vi "FIB trapezoidal mill PXIe-6124.vi"(0 "ActiveX Container":refnum<k7>(container), 1 "COM port":refnum<visa-resource-name>="COM1", 3 "WatchDog Mode":u16(ring)=2 items=["Do Nothing", "Send Idle Only", "Watch FIB & SEM", "Watch FIB Only", "Watch SEM Only"], 5 "FIB Scan Parameters":T3={"X resolution"=512, "Z resolution"=512, "X center"=0.0, "Z center"=0.0, "X size (V)"=20.0, "Z size (V)"=20.0, "Frame line rampdown ratio"=-0.1, "Scan rate (Hz)"=2000000, "Oversampling"=2} {"Z size (V)" min=0.0 max=20.0; "X size (V)" min=0.0 max=20.0; "Frame line rampdown ratio" min=-1.0 max=1.0 step=0.05 format="%.2g"; "Scan rate (Hz)" max=4000000 format="%#.6p"; "Z resolution" max=2048; "X resolution" max=2048}, 7 "FIB HW Config":T4={"FIB X coil"="FIB/ao0", "FIB Y coil"="FIB/ao1", "Beam blank"="FIB/port0/line0", "Ext scan"="FIB/port0/line1", "Detector"="FIB/ai0", "Shutter Drive"="Log/ao0"}, 9 "Options":cluster{"Flip x":bool, "Flip z":bool}={"Flip x"=TRUE, "Flip z"=TRUE}, 11 "Milling para":T1={"X resolution"=4096, "Z resolution"=125001, "X offset (um)"=0.0, "Z offset (um)"=0.0, "X center (um)"=0.0, "Z center (um)"=0.0, "X size (um)"=250.0, "Z size (um)"=250.0, "UL-Ang"=90.0, "UR-Ang"=90.0, "Line milling time (s)"=5.0, "Z-step (nm)"=2.0, "Lines auto pause"=1, "Auto pause"=FALSE, "Mill from Bottom"=FALSE, "FIB FOV (um)"=500.0, "Auto Profile"=FALSE, "Mill start from Last"=FALSE, "FIB PID on"=FALSE, "FIB PID reset"=TRUE, "FIB PID measured"=0, "FIB PID target"=0.0, "FIB PID target slope"=0.0, "FIB PID P"=0.001, "FIB PID I"=0.01, "FIB PID D"=0.0, "Emission (uA)"=1.36, "Suppressor (V)"=50.0, "Auto reheat"=FALSE} caption="Milling Parameters" {"Suppressor (V)" step=0.1 format="%.1g"; "Emission (uA)" step=0.1 format="%.2g"; "FIB PID measured" items=["Spec.", "B.D. 1", "B.D. 2", "Mill", "Spec. +"]; "FIB PID target slope" min=-1 max=1 step=0.1; "UR-Ang" format="%.2f"; "UL-Ang" format="%.2f"; "Z offset (um)" step=0.02 format="%.3g"; "X offset (um)" step=1 format="%.3g"; "FIB FOV (um)" format="%.3g"; "Line milling time (s)" format="%.1f"; "Z center (um)" format="%#.3g"; "X center (um)" format="%#.3g"}, 12 "Machine Type":u8(ring) items=["Feiss", "NVision", "Jeiss"], 14 "Damping":bool) -> (4 "Line progress":u8(slide) scale=0.0..100.0, 6 "Total progress":u8(slide) scale=0.0..100.0, 10 "post-pause lines":u16, 15 "error out":errorcluster)   [LabVIEW 2018]
uses:
  <vilib>/DAQmx/write.llb/DAQmx Write (Analog 2D DBL NChan NSamp).vi
  <vilib>/DAQmx/write.llb/DAQmx Write (Analog 1D DBL 1Chan NSamp).vi
  <vilib>/Analysis/baseanly.llb/Mean (DBL).vi
  <vilib>/DAQmx/write.llb/DAQmx Write (Analog DBL 1Chan 1Samp).vi
  <vilib>/DAQmx/write.llb/DAQmx Write (Analog 1D DBL NChan 1Samp).vi
  <vilib>/DAQmx/create/channels.llb/DAQmx Create Channel (AO-Voltage-Basic).vi
  <vilib>/DAQmx/configure/timing.llb/DAQmx Timing (Sample Clock).vi
  <vilib>/DAQmx/miscellaneous.llb/DAQmx Fill In Error Info.vi
  <vilib>/measure/madcrms.llb/Basic Averaged DC-RMS for 1 Chan.vi
  <vilib>/Analysis/NI_AALBase.lvlib
  <vilib>/measure/NI_MAPro.lvlib
panel:
  out "SEM shutter status":string
  out "Fail #":u8
  out "FIB PID measured":u8
  out "FIB PID on offset":dbl
  out "FIB PID target slope":sgl
  out "FIB PID feedback mean":dbl
  out "FIB PID FB array":dbl[](array[numeric])
  out "Beam blanked":bool=TRUE
  out "FIB PID D":sgl
  out "FIB PID I":sgl
  out "FIB PID P":sgl
  out "FIB PID target":sgl
  out "FIB PID reset":bool
  out "FIB PID on":bool
  out "FIB PID feedback":dbl
  out "UR-Ang":sgl=90.0
  out "UL-Ang":sgl=90.0
  in  "FIB bit size (nm)":dbl
  out "X offset":sgl
  out "Y offset":sgl
  in  "Sweep enabled":bool
  in  "Focus (V)":dbl min=-10.0 max=10.0 step=0.1 format="%.3g"
  in  "Imbalance (V)":dbl min=-10.0 max=10.0 step=0.1 format="%.3f"
  in  "Sweep direction":bool
  in  "Angle (V)":dbl min=-10.0 max=10.0 step=0.1 format="%.3g"
  in  "Position (V)":dbl min=-10.0 max=10.0 step=0.1 format="%.3g"
  in  "Level #":u8
  in  "Sweep #":u8=1 min=1
  out "Shutter Drive":tag="PXI1Slot2/ao0"
  out "Milling mode":T2(ring)=enum."SEM + FIB"
  out "Z voltage RT":dbl
  out "Ext scan":tag="PXI1Slot4/port0/line1"
  out "FIB Y coil":tag="PXI1Slot4/ao1"
  out "FIB X coil":tag="PXI1Slot4/ao0"
  out "Mill from Bottom":bool
  out "Line Paused":bool
  in  "Resume":bool
  in  "Manual pause":bool
  out "Auto pause":bool
  out "Line milling time (s)":sgl=10.0
  out "Lines auto pause":u16=1
  out "Y size":sgl=1.0
  out "X size":sgl=1.0
  out "Y center":sgl
  out "X center":sgl
  out "Y resolution":u32=100
  out "X resolution":u32=16384
  in  "Stop":bool
  out "Beam blank":tag="PXI1Slot4/port0/line0"
  # "% of"
  # "th line"
  # "%"
  # "Direction"
  # "Start\nfrom"
  # "<"
  # "Scan coils"
  # "Flip"
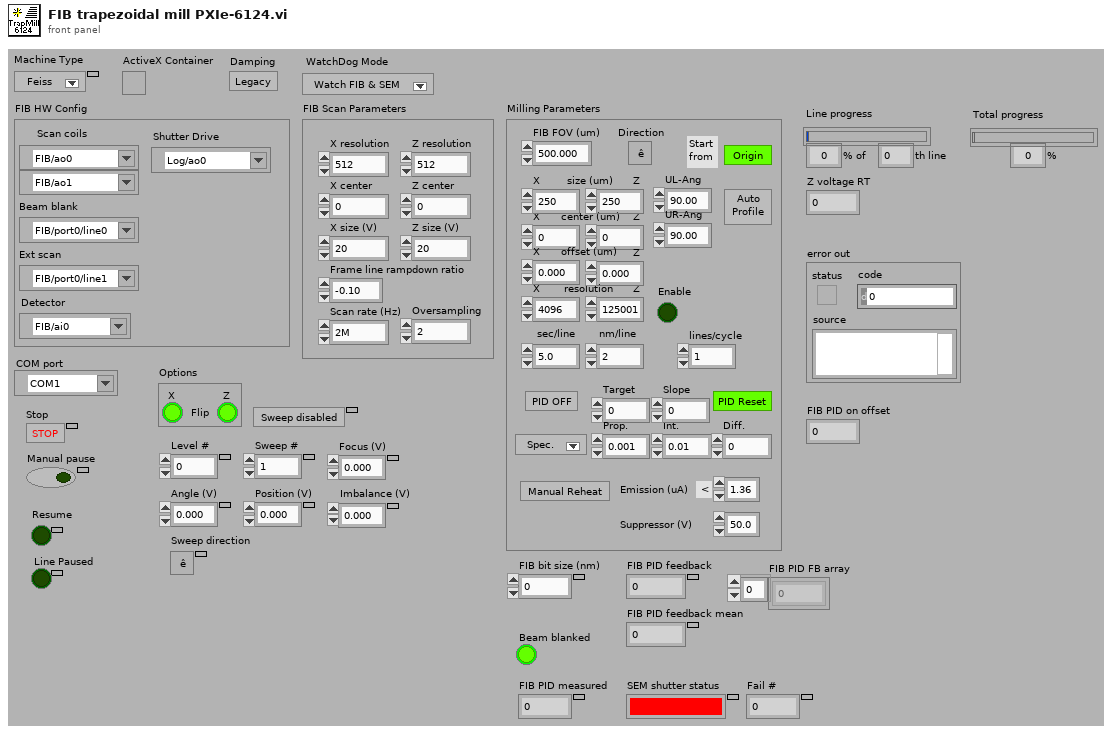
[diagram p1: front panel]
types:
  T1 = cluster{"X resolution":u32, "Z resolution":u32, "X offset (um)":sgl, "Z offset (um)":sgl, "X center (um)":sgl, "Z center (um)":sgl, "X size (um)":sgl, "Z size (um)":sgl, "UL-Ang":sgl, "UR-Ang":sgl, "Line milling time (s)":sgl, "Z-step (nm)":dbl, "Lines auto pause":u16, "Auto pause":bool, "Mill from Bottom":bool, "FIB FOV (um)":sgl, "Auto Profile":bool, "Mill start from Last":bool, "FIB PID on":bool, "FIB PID reset":bool, "FIB PID measured":u8, "FIB PID target":sgl, "FIB PID target slope":sgl, "FIB PID P":sgl, "FIB PID I":sgl, "FIB PID D":sgl, "Emission (uA)":dbl, "Suppressor (V)":sgl, "Auto reheat":bool}
  T2 = enum16{"SEM", "FIB", "Milling", "SEM + FIB", "Mill + SEM", "SEM Drift Correction", "FIB Drift Correction", "No Beam", "External", "External + SEM"}
  T3 = cluster{"X resolution":u32, "Z resolution":u32, "X center":dbl, "Z center":dbl, "X size (V)":dbl, "Z size (V)":dbl, "Frame line rampdown ratio":dbl, "Scan rate (Hz)":u32, "Oversampling":u16}
  T4 = cluster{"FIB X coil":tag, "FIB Y coil":tag, "Beam blank":tag, "Ext scan":tag, "Detector":tag, "Shutter Drive":tag}
  T5 = enum16{"SEM", "FIB", "Mill", "SEM + FIB", "Mill + SEM", "Drift SEM", "Drift FIB", "None", "Ext", "Ext + SEM"}
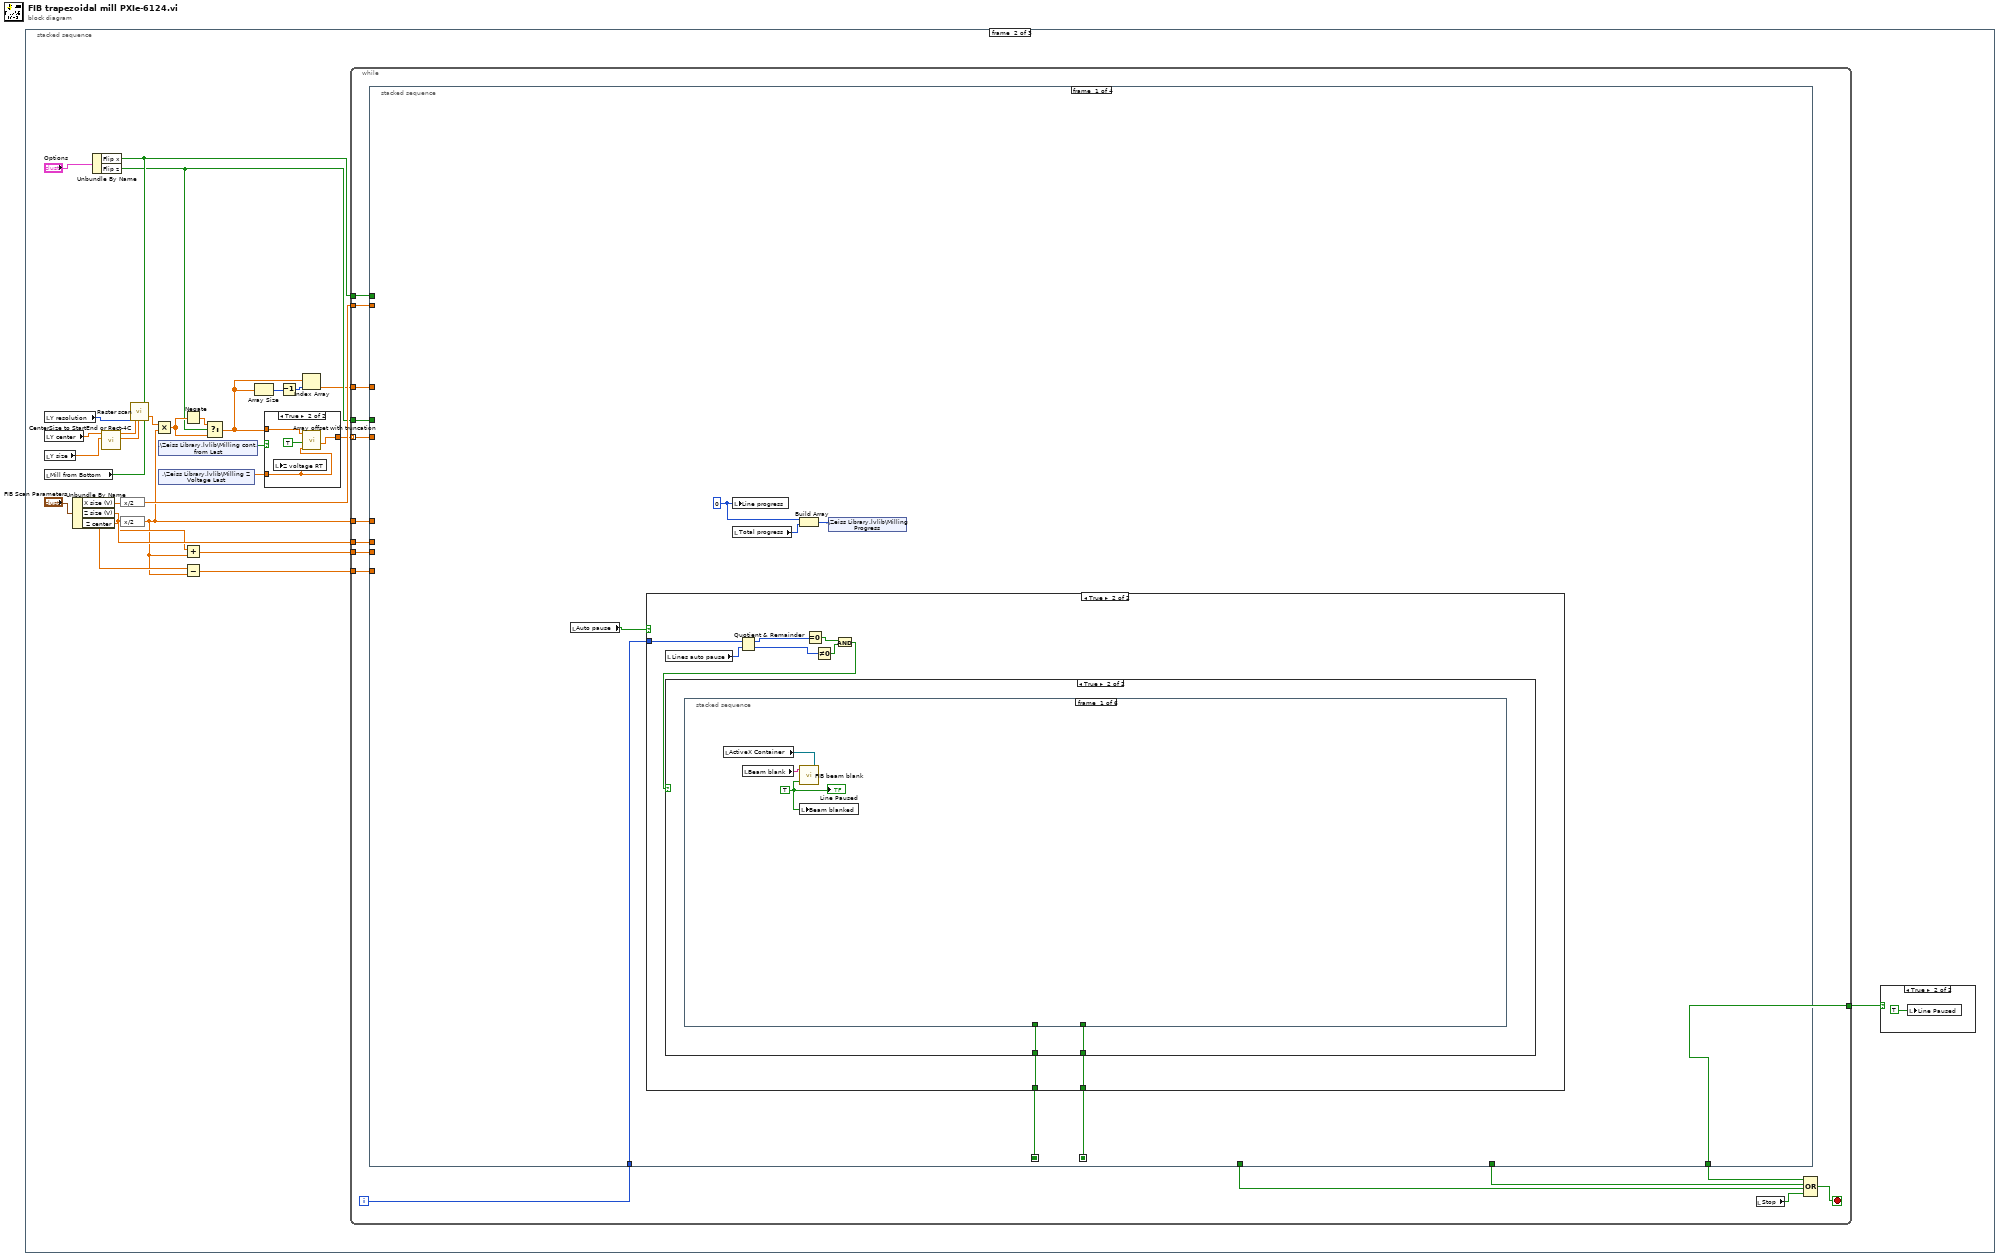
[diagram p0: block diagram]
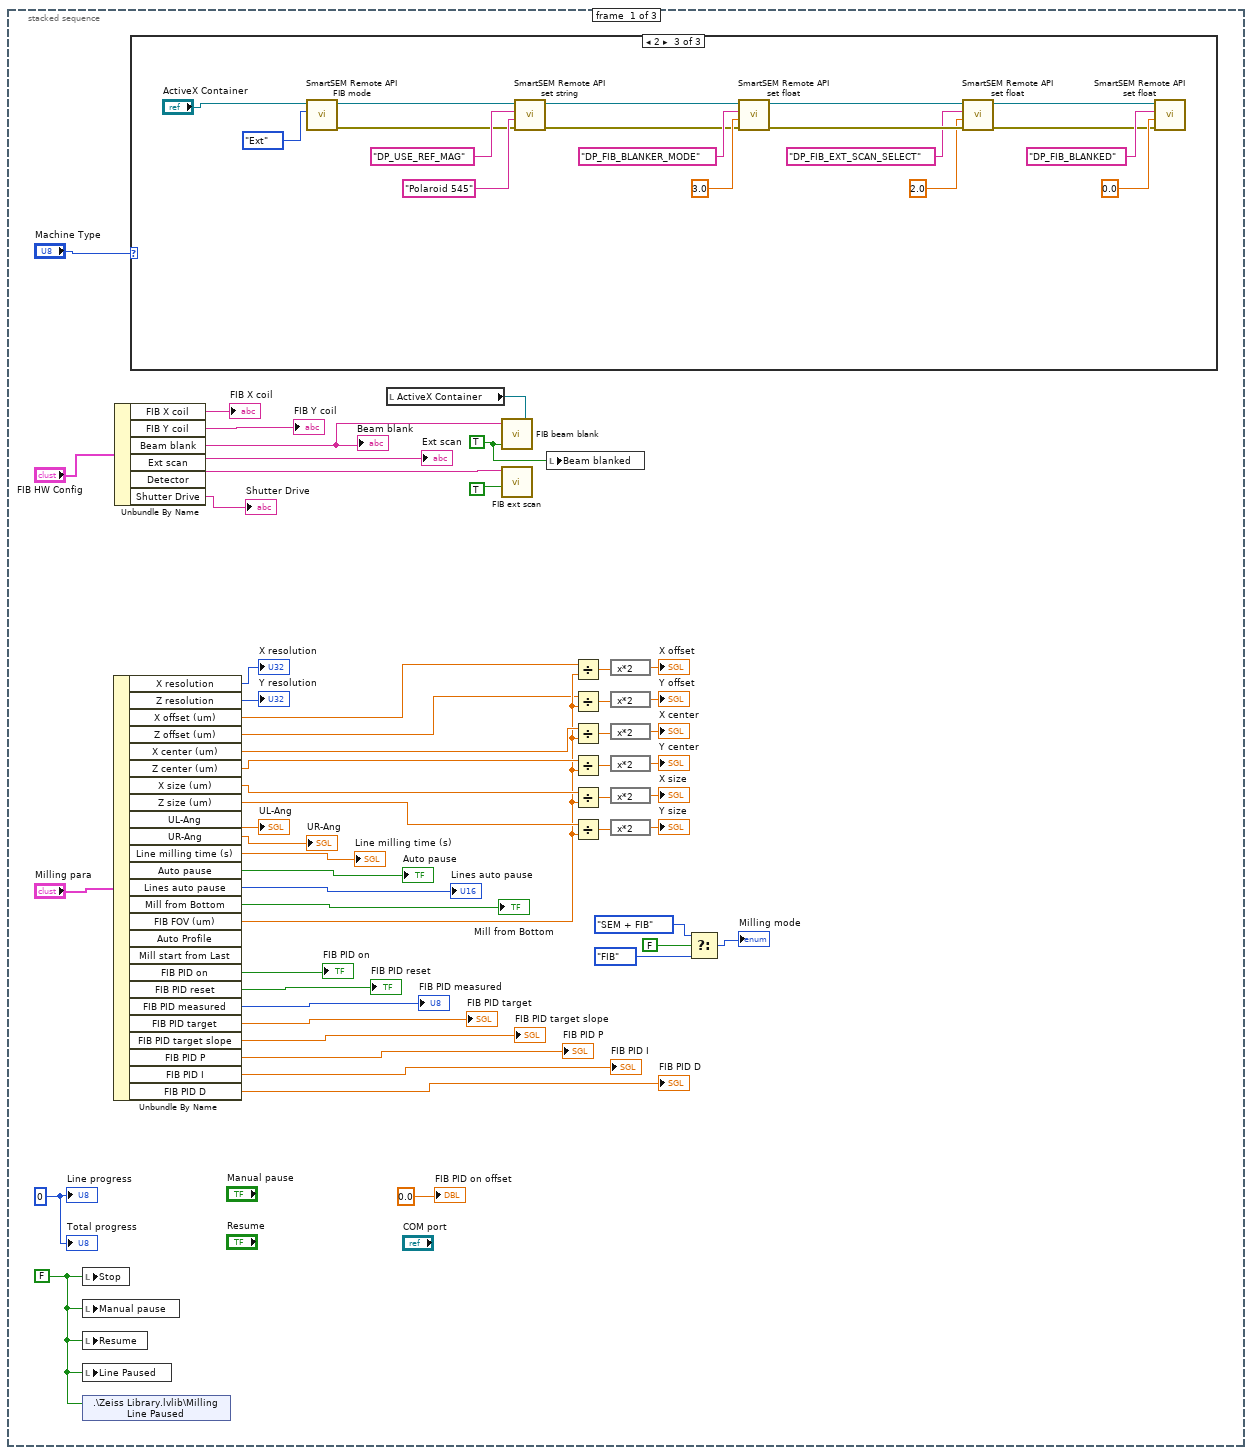
[diagram p2: hidden frame]
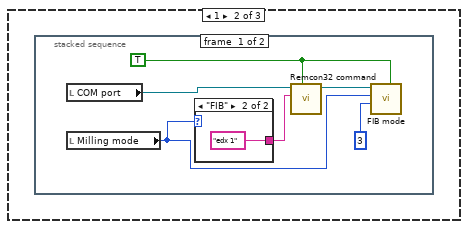
[diagram p4: hidden frame]
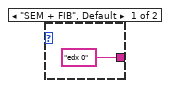
[diagram p5: hidden frame]
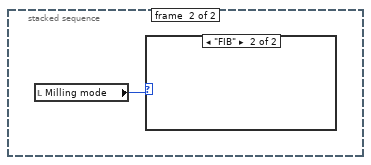
[diagram p6: hidden frame]
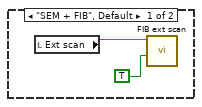
[diagram p7: hidden frame]
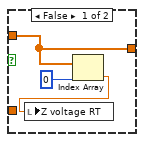
[diagram p8: hidden frame]
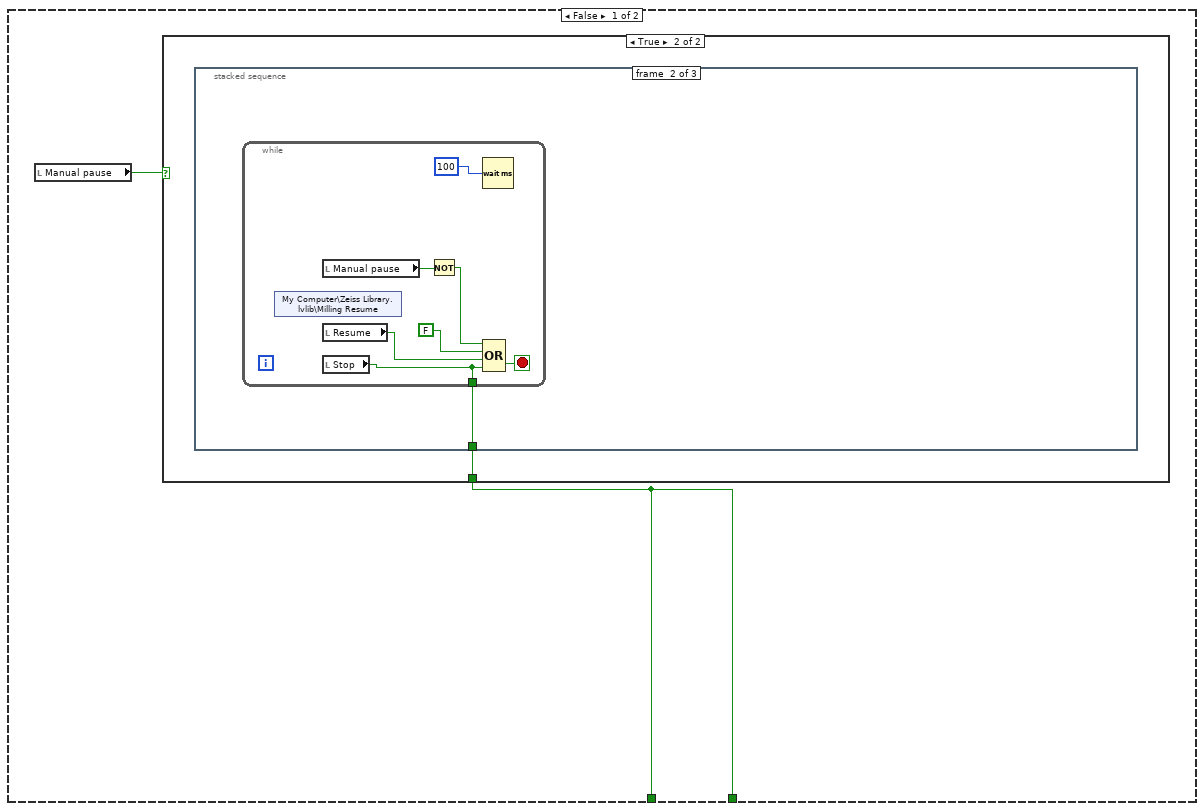
[diagram p10: hidden frame]
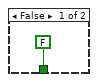
[diagram p11: hidden frame]
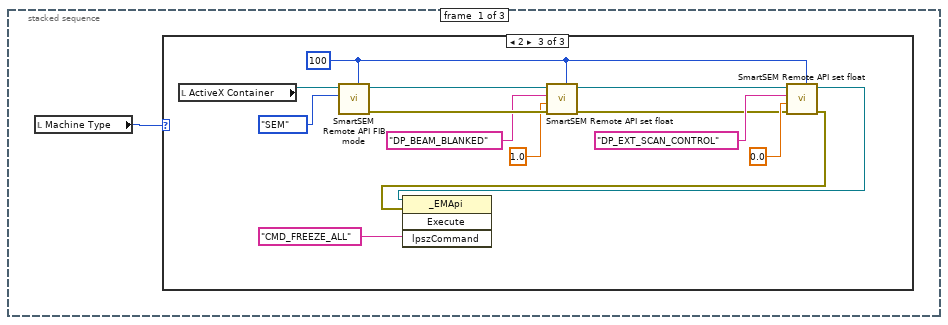
[diagram p12: hidden frame]
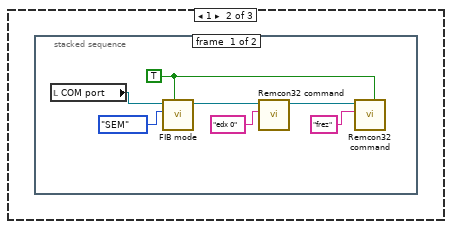
[diagram p14: hidden frame]
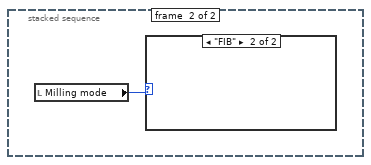
[diagram p15: hidden frame]
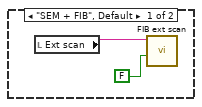
[diagram p16: hidden frame]
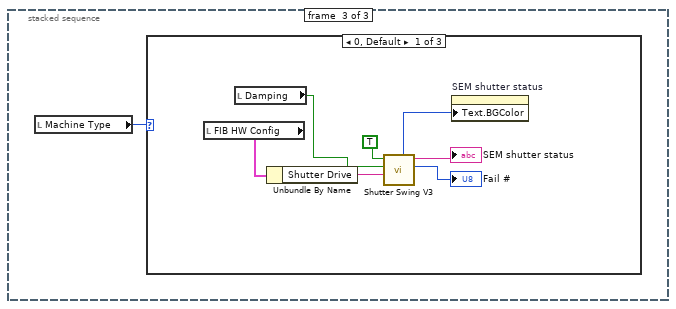
[diagram p17: hidden frame]
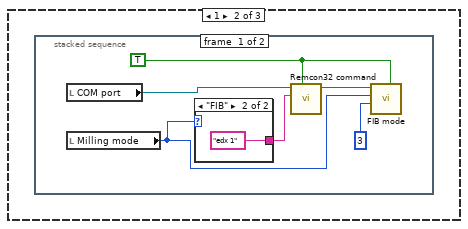
[diagram p18: hidden frame]
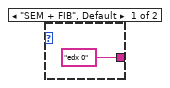
[diagram p19: hidden frame]
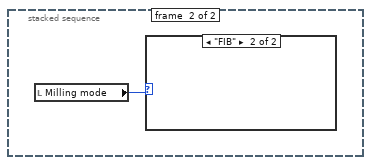
[diagram p20: hidden frame]
diagram:
  n1 = stacked-sequence {
    frame #0 {
      w7 = TRUE ("Beam blanked")
      w43 = FALSE ("Stop")
      w53 = u8 0 ("Milling progress")
      n2 = local write "Stop"(w43) -> ()
      n3 = local write "Manual pause"(w43) -> ()
      n4 = local write "Resume"(w43) -> ()
      n5 = local write "Line Paused"(w43) -> ()
      n6 = shared-variable ".\\Zeiss Library.lvlib\\Milling Line Paused"(w43) -> ()  [unwired: 1 in, 1 out]
      n7 = Unbundle By Name("Milling para") -> ("X resolution"=→"X resolution":u32, "Z resolution"=→"Y resolution":u32, "X offset (um)"=w22:sgl, "Z offset (um)"=w21:sgl, "X center (um)"=w27:sgl, "Z center (um)"=w26:sgl, "X size (um)"=w37:sgl, "Z size (um)"=w33:sgl, "UL-Ang"=→"UL-Ang":sgl, "UR-Ang"=→"UR-Ang":sgl, "Line milling time (s)"=→"Line milling time (s)":sgl, "Auto pause"=→"Auto pause":bool, "Lines auto pause"=→"Lines auto pause":u16, "Mill from Bottom"=→"Mill from Bottom":bool, "FIB FOV (um)"=w23:sgl, "FIB PID on"=→"FIB PID on":bool, "FIB PID reset"=→"FIB PID reset":bool, "FIB PID measured"=→"FIB PID measured":u8, "FIB PID target"=→"FIB PID target":sgl, "FIB PID target slope"=→"FIB PID target slope":sgl, "FIB PID P"=→"FIB PID P":sgl, "FIB PID I"=→"FIB PID I":sgl, "FIB PID D"=→"FIB PID D":sgl)  [unwired: 2 out]
      n8 = Unbundle By Name("FIB HW Config") -> ("FIB X coil"=→"FIB X coil":tag, "FIB Y coil"=→"FIB Y coil":tag, "Beam blank"=w40:tag, "Ext scan"=w41:tag, "Shutter Drive"=→"Shutter Drive":tag)  [unwired: 1 out]
      "Beam blank" <- w40
      "Ext scan" <- w41
      n9 = case shown="2" "Machine Type" {
        frame 0, Default {
        }
        frame 1 {
          n10 = stacked-sequence {
            frame #0 {
              w56 = TRUE ("Initialization")
              n11 = local read "COM port"() -> (w58:refnum<visa-resource-name>)
              n12 = local read "Milling mode"() -> (w54:T2)
              n13 = case shown="\"FIB\"" w54 {
                tunnel: ["edx 0" ("SEM command") "edx 1" ("SEM command")] -> w55
                frame "SEM + FIB", Default {
                }
                frame "FIB" {
                }
              }
              n14 = call "Remcon32 command.vi"("Initialization"=w56, "SEM command"=w55, "COM port in"=w58) -> ("COM port out"=w57:refnum<visa-resource-name>)  [unwired: 5 in, 3 out]
              n15 = call "FIB mode.vi"("Close session"=w56, "Iterations"=u32 3, "FIB mode"=w54, "COM port in"=w57) -> ()  [unwired: 6 in, 2 out]
            }
            frame #1 {
              n16 = local read "Milling mode"() -> (w62:T2)
              n17 = case shown="\"FIB\"" w62 {
                frame "SEM + FIB", Default {
                  n18 = local read "Ext scan"() -> (w63:tag)
                  n19 = call "FIB ext scan.vi"("Ext on"=TRUE ("data"), "FIB Ext Scan"=w63) -> ()  [unwired: 9 in, 1 out]
                }
                frame "FIB" {
                }
              }
            }
          }
        }
        frame 2 {
          n20 = call "SmartSEM Remote API FIB mode.vi"("FIB mode"=T5."Ext", "ActiveX Container"="ActiveX Container") -> ("error out"=w66:errorcluster, "reference out"=w69:refnum<k7>)  [unwired: 8 in]
          n21 = call "SmartSEM Remote API set string.vi"("error in"=w66, "vValue"="Polaroid 545" ("lpszParam"), "lpszParam"="DP_USE_REF_MAG", "ActiveX Container"=w69) -> ("error out"=w67:errorcluster, "reference out"=w68:refnum<k7>)  [unwired: 6 in]
          n22 = call "SmartSEM Remote API set float.vi"("error in"=w67, "vValue"=sgl 3.0, "lpszParam"="DP_FIB_BLANKER_MODE", "ActiveX Container"=w68) -> ("error out"=w76:errorcluster, "reference out"=w77:refnum<k7>)  [unwired: 6 in]
          n23 = call "SmartSEM Remote API set float.vi"("error in"=w76, "vValue"=sgl 2.0, "lpszParam"="DP_FIB_EXT_SCAN_SELECT" ("lpszCommand"), "ActiveX Container"=w77) -> ("error out"=w70:errorcluster, "reference out"=w71:refnum<k7>)  [unwired: 6 in]
          n24 = call "SmartSEM Remote API set float.vi"("error in"=w70, "vValue"=sgl 0.0, "lpszParam"="DP_FIB_BLANKED", "ActiveX Container"=w71) -> ()  [unwired: 6 in, 2 out]
        }
      }
      n25 = local read "ActiveX Container"() -> (w2:refnum<k7>)
      n26 = call "FIB beam blank.vi"("ActiveX Container"=w2, "Beam blanked"=w7, "lines"=w40) -> ()  [unwired: 2 in, 1 out]
      n27 = call "FIB ext scan.vi"("Ext on"=TRUE ("data"), "FIB Ext Scan"=w41) -> ()  [unwired: 9 in, 1 out]
      n28 = local write "Beam blanked"(w7) -> ()
      n29 = Divide(x=w22, y=w23) -> (x/y=w25:sgl)
      n30 = Divide(x=w21, y=w23) -> (x/y=w24:sgl)
      n31 = Divide(x=w27, y=w23) -> (x/y=w30:sgl)
      n32 = Divide(x=w26, y=w23) -> (x/y=w31:sgl)
      n33 = Divide(x=w37, y=w23) -> (x/y=w36:sgl)
      n34 = Divide(x=w33, y=w23) -> (x/y=w34:sgl)
      n35 = expression code="x*2"(w25) -> (→"X offset":sgl)
      n36 = expression code="x*2"(w24) -> (→"Y offset":sgl)
      n37 = expression code="x*2"(w30) -> (→"X center":sgl)
      n38 = expression code="x*2"(w31) -> (→"Y center":sgl)
      n39 = expression code="x*2"(w36) -> (→"X size":sgl)
      n40 = expression code="x*2"(w34) -> (→"Y size":sgl)
      n41 = Select(t=T2."SEM + FIB" ("FIB mode"), s=FALSE, f=T2."FIB" ("FIB mode")) -> (s? t:f=→"Milling mode":T2)
      "Line progress" <- w53
      "Total progress" <- w53
      "FIB PID on offset" <- 0.0 ("FIB PID on offset")
    }
    frame #1 {
      n42 = local read "Y resolution"() -> (w110:u32)
      n43 = local read "Y center"() -> (w109:sgl)
      n44 = local read "Y size"() -> (w102:sgl)
      n45 = local read "Mill from Bottom"() -> (w99:bool)
      n46 = Unbundle By Name("FIB Scan Parameters") -> ("X size (V)"=w103:dbl, "Z size (V)"=w96:dbl, "Z center"=w87:dbl)
      n47 = Unbundle By Name("Options") -> ("Flip x"=w98:bool, "Flip z"=w93:bool)
      n48 = call "CenterSize to StartEnd or Rect-4C.vi"("Size"=w102, "Center"=w109) -> ("End"=w107:dbl, "Start"=w108:dbl)  [unwired: 3 in, 1 out]
      n49 = expression code="x/2"(w103) -> (w97:dbl)
      n50 = expression code="x/2"(w96) -> (w86:dbl)
      n51 = call "Raster scan.vi"("Y resolution"=w110, "Y start"=w108, "Y end"=w107, "Flip x"=w98, "Flip y"=w99) -> ("Y single line pattern"=w100:dbl[])  [unwired: 7 in, 7 out]
      n52 = Multiply(x=w100, y=w86) -> (x*y=w101:dbl[])
      n53 = shared-variable ".\\Zeiss Library.lvlib\\Milling cont. from Last"() -> (w83:bool)  [unwired: 1 in, 1 out]
      n54 = shared-variable ".\\Zeiss Library.lvlib\\Milling Z Voltage Last"() -> (w94:sgl)  [unwired: 1 in, 1 out]
      n55 = Negate(x=w101) -> (-x=w105:dbl[])
      n56 = Add(x=w87, y=w86) -> (x+y=w85:dbl)
      n57 = Subtract(x=w87, y=w86) -> (x-y=w84:dbl)
      n58 = Select(t=w105, s=w93, f=w101) -> (s? t:f=w90:dbl[])
      n59 = Array Size(array=w90) -> (size(s)=w92:i32)
      n60 = case shown="True" w83 {
        tunnel: w90 -> [w113 w116]
        tunnel: [w113 w117] -> w95
        tunnel: w94 -> [_ w114]
        frame False {
          n61 = Index Array(array=w113, index=0) -> (element=w112:dbl)
          n62 = local write "Z voltage RT"(w112) -> ()
        }
        frame True {
          n63 = local write "Z voltage RT"(w114) -> ()
          n64 = call "Array offset with truncation.vi"("New starting value"=w114, "Truncate up"=TRUE, "Input array"=w116) -> ("Truncated array with new starting value"=w117:dbl[])  [unwired: 7 in, 1 out]
        }
      }
      n65 = Decrement(x=w92) -> (x-1=w91:i32)
      n66 = Index Array(array=w90, index=w91) -> (element=w89:dbl)
      n67 = while {
        tunnel: w95 -> [w128] mode=indexing
        tunnel: w98 -> [w131]
        tunnel: w97 -> [w130]
        tunnel: w86 -> [w129]
        tunnel: w96 -> [w127]
        tunnel: w93 -> [w125]
        tunnel: w89 -> [w124]
        tunnel: [w122] -> w88
        tunnel: w85 -> [w121]
        tunnel: w84 -> [w120]
        i -> [w133]
        stop <- w123 stop-if-true
        n68 = stacked-sequence {
          seq-local: [w135 _ _ _] -> [_ _ w316 _]
          seq-local: [w134 _ _ _] -> [_ _ w315 _]
          tunnel: w128 -> [_ _ w319 _]
          tunnel: w133 -> [w139 w309 _ _]
          tunnel: [_ _ w327 _] -> w126
          tunnel: [_ _ w326 _] -> w132
          tunnel: w131 -> [_ _ w321 _]
          tunnel: w130 -> [_ _ w324 _]
          tunnel: w129 -> [_ _ w325 _]
          tunnel: w127 -> [_ _ w322 _]
          tunnel: w125 -> [_ _ w323 _]
          tunnel: w124 -> [_ _ _ _]
          tunnel: [_ _ w320 _] -> w122
          tunnel: w121 -> [_ _ w318 _]
          tunnel: w120 -> [_ _ w317 _]
          frame #0 {
            w136 = u8 0 ("Line progress")
            n69 = local read "Auto pause"() -> (w140:bool)
            n70 = case shown="True" w140 {
              tunnel: w139 -> [_ w210]
              tunnel: [w141 w204] -> w135
              tunnel: [w141 w203] -> w134
              frame False {
                n71 = local read "Manual pause"() -> (w142:bool)
                n72 = case shown="True" w142 {
                  tunnel: [FALSE ("Stop") w144] -> w141
                  frame False {
                  }
                  frame True {
                    n73 = stacked-sequence {
                      tunnel: [_ w170 _] -> w144
                      frame #0 {
                        n74 = local read "Machine Type"() -> (w145:u8)
                        n75 = case shown="2" w145 {
                          frame 0, Default {
                          }
                          frame 1 {
                            n76 = stacked-sequence {
                              frame #0 {
                                w147 = TRUE ("Initialization")
                                n77 = local read "COM port"() -> (w146:refnum<visa-resource-name>)
                                n78 = call "FIB mode.vi"("Initialization"=w147, "FIB mode"=T2."SEM", "COM port in"=w146) -> ("COM port out"=w152:refnum<visa-resource-name>)  [unwired: 7 in, 1 out]
                                n79 = call "Remcon32 command.vi"("SEM command"="edx 0", "COM port in"=w152) -> ("COM port out"=w151:refnum<visa-resource-name>)  [unwired: 6 in, 3 out]
                                n80 = call "Remcon32 command.vi"("Close session"=w147, "SEM command"="frez", "COM port in"=w151) -> ()  [unwired: 5 in, 4 out]
                              }
                              frame #1 {
                                n81 = local read "Milling mode"() -> (w153:T2)
                                n82 = case shown="\"FIB\"" w153 {
                                frame "SEM + FIB", Default {
                                n83 = local read "Ext scan"() -> (w154:tag)
                                n84 = call "FIB ext scan.vi"("Ext on"=FALSE ("data"), "FIB Ext Scan"=w154) -> ()  [unwired: 9 in, 1 out]
                                }
                                frame "FIB" {
                                }
                                }
                              }
                            }
                          }
                          frame 2 {
                            w156 = u32 100 ("wait (ms)")
                            n85 = local read "ActiveX Container"() -> (w167:refnum<k7>)
                            n86 = call "SmartSEM Remote API FIB mode.vi"("Wait (ms)"=w156, "FIB mode"=T5."SEM", "ActiveX Container"=w167) -> ("error out"=w165:errorcluster, "reference out"=w166:refnum<k7>)  [unwired: 7 in]
                            n87 = call "SmartSEM Remote API set float.vi"("wait (ms)"=w156, "error in"=w165, "vValue"=sgl 1.0, "lpszParam"="DP_BEAM_BLANKED", "ActiveX Container"=w166) -> ("error out"=w159:errorcluster, "reference out"=w160:refnum<k7>)  [unwired: 5 in]
                            n88 = call "SmartSEM Remote API set float.vi"("wait (ms)"=w156, "error in"=w159, "vValue"=sgl 0.0, "lpszParam"="DP_EXT_SCAN_CONTROL" ("lpszCommand"), "ActiveX Container"=w160) -> ("error out"=w157:errorcluster, "reference out"=w158:refnum<k7>)  [unwired: 5 in]
                            n89 = invoke class="_EMApi" method="Execute"(reference=w158, error in=w157, "lpszCommand"="CMD_FREEZE_ALL") -> ()  [unwired: 1 in, 4 out]
                          }
                        }
                      }
                      frame #1 {
                        n90 = while {
                          tunnel: [w171] -> w170
                          stop <- w176 stop-if-true
                          n91 = shared-variable "My Computer\\Zeiss Library.lvlib\\Milling Resume"() -> ()  [unwired: 1 in, 2 out]
                          n92 = local read "Manual pause"() -> (w174:bool)
                          n93 = local read "Resume"() -> (w175:bool)
                          n94 = local read "Stop"() -> (w171:bool)
                          n95 = Not(x=w174) -> (.not. x?=w173:bool)
                          n96 = Wait (ms)(milliseconds to wait=u32 100) -> ()  [unwired: 1 out]
                          n97 = Compound Arithmetic op=OR(w173, FALSE ("value"), w175, w171) -> (w176:bool)
                        }
                      }
                      frame #2 {
                        n98 = local read "Machine Type"() -> (w178:u8)
                        n99 = case shown="0, Default" w178 {
                          frame 0, Default {
                            n100 = local read "FIB HW Config"() -> (w182:T4)
                            n101 = local read "Damping"() -> (w179:bool)
                            n102 = Unbundle By Name(w182) -> ("Shutter Drive"=w181:tag)
                            n103 = call "Shutter Swing V3.vi"("Shutter Drive"=w181, "Damping"=w179, "Shutter close"=TRUE) -> ("Fail #"=→"Fail #":u8, "SEM shutter status"=→"SEM shutter status":string, "Color Box"=w180:u32)  [unwired: 2 in, 4 out]
                            n104 = property on="SEM shutter status" class="Str"("Text.BGColor"=w180) -> ()  [unwired: 2 in, 2 out]
                          }
                          frame 1 {
                            n105 = stacked-sequence {
                              frame #0 {
                                w188 = TRUE ("Initialization")
                                n106 = local read "COM port"() -> (w190:refnum<visa-resource-name>)
                                n107 = local read "Milling mode"() -> (w186:T2)
                                n108 = case shown="\"FIB\"" w186 {
                                tunnel: ["edx 0" ("SEM command") "edx 1" ("SEM command")] -> w187
                                frame "SEM + FIB", Default {
                                }
                                frame "FIB" {
                                }
                                }
                                n109 = call "Remcon32 command.vi"("Initialization"=w188, "SEM command"=w187, "COM port in"=w190) -> ("COM port out"=w189:refnum<visa-resource-name>)  [unwired: 5 in, 3 out]
                                n110 = call "FIB mode.vi"("Close session"=w188, "Iterations"=u32 3, "FIB mode"=w186, "COM port in"=w189) -> ()  [unwired: 6 in, 2 out]
                              }
                              frame #1 {
                                n111 = local read "Milling mode"() -> (w194:T2)
                                n112 = case shown="\"FIB\"" w194 {
                                frame "SEM + FIB", Default {
                                n113 = local read "Ext scan"() -> (w195:tag)
                                n114 = call "FIB ext scan.vi"("Ext on"=TRUE ("data"), "FIB Ext Scan"=w195) -> ()  [unwired: 9 in, 1 out]
                                }
                                frame "FIB" {
                                }
                                }
                              }
                            }
                          }
                          frame 2 {
                            n115 = local read "ActiveX Container"() -> (w199:refnum<k7>)
                            n116 = call "SmartSEM Remote API FIB mode.vi"("FIB mode"=T5."Ext", "ActiveX Container"=w199) -> ("error out"=w197:errorcluster, "reference out"=w198:refnum<k7>)  [unwired: 8 in]
                            n117 = invoke class="_EMApi" method="Set"(reference=w198, error in=w197, "lpszParam"="DP_FIB_BLANKED", "vValue"=sgl 0.0) -> ()  [unwired: 1 in, 5 out]
                          }
                        }
                      }
                    }
                  }
                }
              }
              frame True {
                n118 = local read "Lines auto pause"() -> (w205:u16)
                n119 = Quotient & Remainder(x=w210, y=w205) -> (x-y*floor(x/y)=w211:i32, floor(x/y)=w209:i32)
                n120 = Equal To 0?(x=w211) -> (x = 0?=w207:bool)
                n121 = Not Equal To 0?(x=w209) -> (x != 0?=w208:bool)
                n122 = And(x=w207, y=w208) -> (x .and. y?=w206:bool)
                n123 = case shown="True" w206 {
                  tunnel: [w212 w215] -> w204
                  tunnel: [w212 w214] -> w203
                  frame False {
                    w212 = FALSE ("Stop")
                    n124 = local write "FIB PID reset"(TRUE ("FIB PID reset")) -> ()
                  }
                  frame True {
                    n125 = stacked-sequence {
                      tunnel: [_ w219 _ _ _ _] -> w215
                      tunnel: [_ _ _ w238 _ _] -> w214
                      frame #0 {
                        w217 = TRUE ("Beam blanked")
                        n126 = local read "ActiveX Container"() -> (w216:refnum<k7>)
                        n127 = local read "Beam blank"() -> (w218:tag)
                        n128 = call "FIB beam blank.vi"("ActiveX Container"=w216, "Beam blanked"=w217, "lines"=w218) -> ()  [unwired: 2 in, 1 out]
                        n129 = local write "Beam blanked"(w217) -> ()
                        "Line Paused" <- w217
                      }
                      frame #1 {
                        n130 = local read "Machine Type"() -> (w220:u8)
                        n131 = while {
                          tunnel: w220 -> [w222]
                          tunnel: [w221] -> w219
                          stop <- w223 stop-if-true
                          n132 = case shown="0, Default" w222 {
                            frame 1 {
                            }
                            frame 0, Default {
                              n133 = shared-variable ".\\Zeiss Library.lvlib\\Logs"() -> (w233:sgl[])  [unwired: 1 in, 1 out]
                              n134 = shared-variable ".\\Zeiss Library.lvlib\\Faraday cup offset"() -> (w229:sgl)  [unwired: 1 in, 1 out]
                              n135 = Index Array(array=w233, index=0) -> (element=w227:sgl)
                              n136 = Subtract(x=w227, y=w229) -> (x-y=w228:sgl)
                              n137 = Less?(x=w228, y=sgl 0.1) -> (x < y?=w230:bool)
                              n138 = case shown="True" w230 {
                                frame False {
                                }
                                frame True {
                                n139 = local read "ActiveX Container"() -> (w234:refnum<k7>)
                                n140 = local read "Beam blank"() -> (w236:tag)
                                n141 = call "FIB beam blank.vi"("ActiveX Container"=w234, "Beam blanked"=TRUE, "lines"=w236) -> ()  [unwired: 2 in, 1 out]
                                }
                              }
                            }
                          }
                          n142 = Wait Until Next ms Multiple(millisecond multiple=u32 100 ("milliseconds to wait")) -> ()  [unwired: 1 out]
                          n143 = shared-variable "My Computer\\Zeiss Library.lvlib\\Milling Resume"() -> (w224:bool)  [unwired: 1 in, 1 out]
                          n144 = local read "Resume"() -> (w225:bool)
                          n145 = local read "Stop"() -> (w221:bool)
                          n146 = Compound Arithmetic op=OR(w224, w225, w221) -> (w223:bool)
                        }
                      }
                      frame #2 {
                        w237 = FALSE ("Resume")
                        n147 = local write "Resume"(w237) -> ()
                        n148 = shared-variable "My Computer\\Zeiss Library.lvlib\\Milling Resume"(w237) -> ()  [unwired: 1 in, 1 out]
                        n149 = local write "Line Paused"(w237) -> ()
                      }
                      frame #3 {
                        n150 = local read "Manual pause"() -> (w239:bool)
                        n151 = case shown="True" w239 {
                          tunnel: [FALSE ("Stop") w241] -> w238
                          frame False {
                          }
                          frame True {
                            n152 = stacked-sequence {
                              seq-local: [w242 _ _] -> [_ _ w250]
                              tunnel: [w242 _ _] -> w241
                              frame #0 {
                                n153 = while {
                                tunnel: [w243] -> w242
                                stop <- w247 stop-if-true
                                n154 = local read "Manual pause"() -> (w245:bool)
                                n155 = Wait Until Next ms Multiple(millisecond multiple=u32 100 ("milliseconds to wait")) -> ()  [unwired: 1 out]
                                n156 = local read "Resume"() -> (w244:bool)
                                n157 = local read "Stop"() -> (w243:bool)
                                n158 = Not(x=w245) -> (.not. x?=w246:bool)
                                n159 = Compound Arithmetic op=OR(w246, w244, w243) -> (w247:bool)
                                }
                              }
                              frame #1 {
                                n160 = shared-variable ".\\Zeiss Library.lvlib\\Milling Z Voltage Last"() -> (w249:sgl)  [unwired: 1 in, 1 out]
                                n161 = local write "Z voltage RT"(w249) -> ()
                              }
                              frame #2 {
                                n162 = case shown="False" w250 {
                                frame False {
                                n163 = local read "Machine Type"() -> (w251:u8)
                                n164 = case shown="2" w251 {
                                frame 0, Default {
                                }
                                frame 1 {
                                n165 = stacked-sequence {
                                frame #0 {
                                w254 = TRUE ("Initialization")
                                n166 = local read "COM port"() -> (w256:refnum<visa-resource-name>)
                                n167 = local read "Milling mode"() -> (w252:T2)
                                n168 = case shown="\"FIB\"" w252 {
                                tunnel: ["edx 0" ("SEM command") "edx 1" ("SEM command")] -> w253
                                frame "SEM + FIB", Default {
                                }
                                frame "FIB" {
                                }
                                }
                                n169 = call "Remcon32 command.vi"("Initialization"=w254, "SEM command"=w253, "COM port in"=w256) -> ("COM port out"=w255:refnum<visa-resource-name>)  [unwired: 5 in, 3 out]
                                n170 = call "FIB mode.vi"("Close session"=w254, "Iterations"=u32 3, "FIB mode"=w252, "COM port in"=w255) -> ()  [unwired: 6 in, 2 out]
                                }
                                frame #1 {
                                n171 = local read "Milling mode"() -> (w260:T2)
                                n172 = case shown="\"SEM + FIB\", Default" w260 {
                                frame "SEM + FIB", Default {
                                n173 = local read "Ext scan"() -> (w261:tag)
                                n174 = call "FIB ext scan.vi"("Ext on"=TRUE ("data"), "FIB Ext Scan"=w261) -> ()  [unwired: 9 in, 1 out]
                                }
                                frame "FIB" {
                                }
                                }
                                }
                                }
                                }
                                frame 2 {
                                w276 = u32 100 ("wait (ms)")
                                n175 = local read "ActiveX Container"() -> (w273:refnum<k7>)
                                n176 = call "SmartSEM Remote API FIB mode.vi"("Wait (ms)"=w276, "FIB mode"=T5."SEM", "ActiveX Container"=w273) -> ("error out"=w271:errorcluster, "reference out"=w272:refnum<k7>)  [unwired: 7 in]
                                n177 = call "SmartSEM Remote API set float.vi"("wait (ms)"=w276, "error in"=w271, "vValue"=sgl 1.0, "lpszParam"="DP_BEAM_BLANKED", "ActiveX Container"=w272) -> ("error out"=w265:errorcluster, "reference out"=w266:refnum<k7>)  [unwired: 5 in]
                                n178 = call "SmartSEM Remote API set float.vi"("wait (ms)"=w276, "error in"=w265, "vValue"=sgl 0.0, "lpszParam"="DP_EXT_SCAN_CONTROL" ("lpszCommand"), "ActiveX Container"=w266) -> ("error out"=w263:errorcluster, "reference out"=w264:refnum<k7>)  [unwired: 5 in]
                                n179 = invoke class="_EMApi" method="Execute"(reference=w264, error in=w263, "lpszCommand"="CMD_FREEZE_ALL") -> ()  [unwired: 1 in, 4 out]
                                }
                                }
                                }
                                frame True {
                                }
                                }
                              }
                            }
                          }
                        }
                      }
                      frame #4 {
                        n180 = local read "FIB HW Config"() -> (w282:T4)
                        n181 = Unbundle By Name(w282) -> ("Shutter Drive"=w277:tag)
                        n182 = local read "Damping"() -> (w278:bool)
                        n183 = call "Shutter Swing V3.vi"("Shutter Drive"=w277, "Damping"=w278, "Shutter close"=TRUE) -> ("Fail #"=w280:u8, "SEM shutter status"=w281:string, "Color Box"=w279:u32)  [unwired: 2 in, 4 out]
                        n184 = property on="SEM shutter status" class="Str"("Text.BGColor"=w279) -> ()  [unwired: 2 in, 2 out]
                        n185 = local write "SEM shutter status"(w281) -> ()
                        n186 = local write "Fail #"(w280) -> ()
                      }
                      frame #5 {
                        n187 = local read "Stop"() -> (w284:bool)
                        n188 = case shown="False" w284 {
                          frame False {
                            n189 = local read "Machine Type"() -> (w285:u8)
                            n190 = case shown="2" w285 {
                              frame 0, Default {
                              }
                              frame 1 {
                                n191 = stacked-sequence {
                                frame #0 {
                                w288 = TRUE ("Initialization")
                                n192 = local read "COM port"() -> (w290:refnum<visa-resource-name>)
                                n193 = local read "Milling mode"() -> (w286:T2)
                                n194 = case shown="\"FIB\"" w286 {
                                tunnel: ["edx 0" ("SEM command") "edx 1" ("SEM command")] -> w287
                                frame "SEM + FIB", Default {
                                }
                                frame "FIB" {
                                }
                                }
                                n195 = call "Remcon32 command.vi"("Initialization"=w288, "SEM command"=w287, "COM port in"=w290) -> ("COM port out"=w289:refnum<visa-resource-name>)  [unwired: 5 in, 3 out]
                                n196 = call "FIB mode.vi"("Close session"=w288, "Iterations"=u32 3, "FIB mode"=w286, "COM port in"=w289) -> ()  [unwired: 6 in, 2 out]
                                }
                                frame #1 {
                                n197 = local read "Milling mode"() -> (w294:T2)
                                n198 = case shown="\"FIB\"" w294 {
                                frame "SEM + FIB", Default {
                                n199 = local read "Ext scan"() -> (w295:tag)
                                n200 = call "FIB ext scan.vi"("Ext on"=TRUE ("data"), "FIB Ext Scan"=w295) -> ()  [unwired: 9 in, 1 out]
                                }
                                frame "FIB" {
                                }
                                }
                                }
                                }
                              }
                              frame 2 {
                                n201 = local read "ActiveX Container"() -> (w305:refnum<k7>)
                                n202 = call "SmartSEM Remote API FIB mode.vi"("FIB mode"=T5."Ext", "ActiveX Container"=w305) -> ("error out"=w299:errorcluster, "reference out"=w302:refnum<k7>)  [unwired: 8 in]
                                n203 = call "SmartSEM Remote API set float.vi"("error in"=w299, "vValue"=sgl 0.0, "lpszParam"="DP_FIB_BLANKED", "ActiveX Container"=w302) -> ("error out"=w300:errorcluster, "reference out"=w301:refnum<k7>)  [unwired: 6 in]
                                n204 = call "SmartSEM Remote API detectors.vi"("error in"=w300, "Det A Type"="InLens", "ActiveX Container"=w301) -> ()  [unwired: 7 in, 2 out]
                              }
                            }
                          }
                          frame True {
                          }
                        }
                      }
                    }
                  }
                }
              }
            }
            n205 = local write "Line progress"(w136) -> ()
            n206 = local read "Total progress"() -> (w138:u8)
            n207 = Build Array(w136, w138) -> (w137:u8[])
            n208 = shared-variable ".\\Zeiss Library.lvlib\\Milling Progress"(w137) -> ()  [unwired: 1 in, 1 out]
          }
          frame #1 {
            n209 = local read "Machine Type"() -> (w306:u8)
            n210 = local read "Lines auto pause"() -> (w310:u16)
            n211 = case shown="2" w306 {
              frame 0, Default {
              }
              frame 2 {
                n212 = local read "ActiveX Container"() -> (w312:refnum<k7>)
                n213 = shared-variable "My Computer\\Zeiss Library.lvlib\\FIB FOV (um)"() -> (w313:sgl)  [unwired: 1 in, 1 out]
                n214 = call "SmartSEM Remote API FIB mag.vi"("FIB FOV (um)"=w313, "ActiveX Container"=w312) -> ()  [unwired: 8 in, 2 out]
              }
            }
            n215 = Quotient & Remainder(x=w309, y=w310) -> (x-y*floor(x/y)=w311:i32)  [unwired: 1 out]
            n216 = Increment(x=w311) -> (x+1=w308:i32)
            "post-pause lines" <- w308
            n217 = local write "FIB PID FB array"(dbl[] [] ("FIB PID FB array")) -> ()
            n218 = shared-variable ".\\Zeiss Library.lvlib\\Milling Post-pause Lines"(w308) -> ()  [unwired: 1 in, 1 out]
          }
          frame #2 {
            n219 = Or(x=w315, y=w316) -> (x .or. y?=w314:bool)
            n220 = case shown="False" w314 {
              tunnel: [w466 w771] -> w327
              tunnel: [w462 w771] -> w326
              tunnel: w325 -> [w440 _]
              tunnel: w324 -> [w420 _]
              tunnel: w323 -> [w414 _]
              tunnel: w322 -> [w412 _]
              tunnel: w321 -> [w409 _]
              tunnel: [w394 w771] -> w320
              tunnel: w319 -> [w388 _]
              tunnel: w318 -> [w386 _]
              tunnel: w317 -> [w385 _]
              frame False {
                w359 = -0.01 ("x")
                w399 = -0.1 ("x")
                w461 = 10123 items=["Finite Samples"=10178, "Continuous Samples"=10123, "Hardware Timed Single Point"=12522] ("sample mode")
                # "Watch for \nFIB HOME"
                # "Watch FIB Scan\n(or early Home)"
                n221 = local read "Milling para"() -> (w393:T1)
                n222 = Unbundle By Name(w393) -> ("X size (um)"=w407:sgl, "FIB FOV (um)"=w383:sgl)
                n223 = local read "Z voltage RT"() -> (w328:dbl)
                n224 = local read "FIB PID on"() -> (w391:bool)
                n225 = local read "FIB PID on offset"() -> (w387:dbl)
                n226 = local read "X resolution"() -> (w419:u32)
                n227 = Add(x=w388, y=w387) -> (x+y=w389:dbl)
                n228 = local read "Machine Type"() -> (w418:u8)
                n229 = local read "FIB X coil"() -> (w464:tag)
                n230 = local read "FIB Y coil"() -> (w463:tag)
                n231 = Select(t=w328, s=w391, f=w389) -> (s? t:f=w390:dbl)
                n232 = Negate(x=w390) -> (-x=w415:dbl)
                n233 = Select(t=w415, s=w414, f=w390) -> (s? t:f=w413:dbl)
                n234 = Divide(x=w413, y=w412) -> (x/y=w410:dbl)
                n235 = Multiply(x=w383, y=w410) -> (x*y=w411:dbl)
                n236 = call "Milling parameter to trapezoidal shape.vi"("Y location (um)"=w411, "Milling para"=w393) -> ("X end"=w416:dbl, "X start"=w417:dbl, "X size (um) @ Y"=w408:dbl, "Total progress"=w396:dbl)  [unwired: 5 in, 1 out]
                n237 = call "Raster scan.vi"("X resolution"=w419, "Frame line rampdown ratio"=0.0, "X start"=w417, "X end"=w416, "Flip x"=w409) -> ("X resolution with rampdown"=w422:i32, "X single line pattern"=w425:dbl[])  [unwired: 7 in, 6 out]
                n238 = case shown="True" "Sweep enabled" {
                  tunnel: [_ w491] -> w449
                  tunnel: [_ w490] -> w448
                  frame False {
                  }
                  frame True {
                    w498 = 10123 items=["Finite Samples"=10178, "Continuous Samples"=10123, "Hardware Timed Single Point"=12522] ("sample mode")
                    n239 = local read "Line milling time (s)"() -> (w496:sgl)
                    n240 = local read "Shutter Drive"() -> (w488:tag)
                    n241 = call "Beam deflector.vi"("Sweep direction"="Sweep direction", "Level #"="Level #", "Imbalance (V)"="Imbalance (V)", "Position (V)"="Position (V)", "Angle (V)"="Angle (V)", "Focus (V)"="Focus (V)") -> ("All posts"=w477:dbl[][])  [unwired: 5 in]
                    n242 = call-poly <vilib>:"DAQmx Create Virtual Channel.vi"("physical channels"=w488) -> ("task out"=w476:refnum<k21>, "error out"=w475:errorcluster)  [unwired: 13 in]
                    n243 = Multiply(x="Level #", y="Sweep #") -> (x*y=w484:u8)
                    n244 = In Range and Coerce(upper limit=u8 255 ("lower limit"), x=w484, lower limit=u8 1) -> (coerced(x)=w485:u8)  [unwired: 1 out]
                    n245 = Divide(x=w485, y=w496) -> (x/y=w497:sgl)
                    n246 = call-poly <vilib>:"DAQmx Timing.vi"("task/channels in"=w476, "sample mode"=w498, "rate"=w497, "error in"=w475) -> ("task out"=w493:refnum<k21>, "error out"=w492:errorcluster)  [unwired: 3 in, 7 out]
                    n247 = call-poly <vilib>:"DAQmx Write.vi"("task/channels in"=w493, "data"=w477, "error in"=w492) -> ("task out"=w494:refnum<k21>, "error out"=w495:errorcluster)  [unwired: 1 in, 10 out]
                    n248 = call <vilib>:"DAQmx Start Task.vi"("task/channels in"=w494, "error in"=w495) -> ("task out"=w491:refnum<k21>, "error out"=w490:errorcluster)  [unwired: 12 in]
                  }
                }
                n249 = Divide(x=w408, y=w407) -> (x/y=w406:dbl)
                n250 = Multiply(x=w425, y=w420) -> (x*y=w427:dbl[])
                n251 = expression code="1e6/x"(w419) -> (w429:u32)
                n252 = Negate(x=w427) -> (-x=w426:dbl[])
                n253 = Round Toward +Infinity(x=w429) -> (ceil(x): smallest int >= x=w430:u32)
                n254 = Select(t=w426, s=w409, f=w427) -> (s? t:f=w424:dbl[])
                n255 = case shown="2" w418 {
                  tunnel: [5.0 ("minimum value") 10.0 ("minimum value") 8.0 ("minimum value")] -> w354
                  tunnel: [-5.0 ("minimum value") -10.0 ("minimum value") -8.0 ("minimum value")] -> w353
                  frame 0, Default {
                  }
                  frame 1 {
                  }
                  frame 2 {
                  }
                }
                n256 = call-poly <vilib>:"DAQmx Create Virtual Channel.vi"("maximum value"=w354, "minimum value"=w353, "physical channels"=w464) -> ("task out"=w439:refnum<k21>, "error out"=w438:errorcluster)  [unwired: 6 in, 5 out]
                n257 = call-poly <vilib>:"DAQmx Create Virtual Channel.vi"("maximum value"=w354, "minimum value"=w353, "physical channels"=w463) -> ("task out"=w437:refnum<k21>, "error out"=w436:errorcluster)  [unwired: 6 in, 5 out]
                n258 = Less Or Equal?(x=100.0, y=w396) -> (x <= y?=w394:bool)
                n259 = Divide(x=sgl 0.2, y=w383) -> (x/y=w380:sgl)
                n260 = for {
                  N: w430 -> [_]
                  tunnel: w424 -> [w470]
                  tunnel: [w470] -> w423 mode=indexing
                }
                n261 = Multiply(x=w430, y=w422) -> (x*y=w431:u32)
                n262 = Random Number (0-1)() -> (number: 0 to 1=w381:dbl)
                n263 = local read "Milling para"() -> (w402:T1)
                n264 = local read "Options"() -> (w403:cluster{"Flip x":bool, "Flip z":bool})
                n265 = Reshape Array(w423, w431) -> (w428:dbl[])
                n266 = Multiply(x=w381, y=w380) -> (x*y=w379:dbl)
                n267 = local read "X offset"() -> (w378:sgl)
                n268 = local read "Y offset"() -> (w442:sgl)
                n269 = Round Toward -Infinity(1:w396) -> (0:w397:dbl)
                n270 = Add(x=w379, y=w378) -> (x+y=w377:dbl)
                n271 = Unbundle By Name(w402) -> ("Mill from Bottom"=w404:bool)
                n272 = Unbundle By Name(w403) -> ("Flip z"=w405:bool)
                n273 = Multiply(x=w377, y=w420) -> (x*y=w443:dbl)
                n274 = Multiply(x=w442, y=w440) -> (x*y=w441:dbl)
                n275 = call-poly <vilib>:"DAQmx Timing.vi"("task/channels in"=w439, "sample mode"=w461, "rate"=1000000.0 ("Milling rate"), "error in"=w438) -> ("task out"=w456:refnum<k21>, "error out"=w455:errorcluster)  [unwired: 3 in, 7 out]
                n276 = To Unsigned Byte Integer(number=w397) -> (unsigned 8bit integer=w398:u8)
                n277 = shared-variable ".\\Zeiss Library.lvlib\\Faraday Cup before mill"() -> (w351:sgl)  [unwired: 1 in, 1 out]
                n278 = Negate(x=w443) -> (-x=w444:dbl)
                n279 = Negate(x=w441) -> (-x=w446:dbl)
                n280 = Select(t=w444, s=w409, f=w443) -> (s? t:f=w445:dbl)
                n281 = Select(t=w446, s=w414, f=w441) -> (s? t:f=w392:dbl)
                n282 = Exclusive Or(1:w405, 2:w404) -> (0:w357:bool)
                n283 = Compound Arithmetic op=ADD(w445, w428) -> (w355:dbl[])
                n284 = In Range and Coerce(upper limit=w354, x=w355, lower limit=w353) -> (coerced(x)=w352:dbl[])  [unwired: 1 out]
                n285 = Add(x=w390, y=w392) -> (x+y=w432:dbl)
                n286 = call-poly <vilib>:"DAQmx Write.vi"("task/channels in"=w456, "data"=w352, "error in"=w455) -> ("task out"=w454:refnum<k21>, "error out"=w335:errorcluster)  [unwired: 1 in, 10 out]
                n287 = Negate(x=w399) -> (-x=w400:dbl)
                n288 = Negate(x=w359) -> (-x=w358:dbl)
                n289 = call "FM Gen Pulse for FIB-SEM.vi"("WatchDog Mode"="WatchDog Mode", "error in"=w335, "State Value"=i16 2) -> ()  [unwired: 6 in, 3 out]
                n290 = expression code="x/20"(w351) -> (w350:sgl)
                n291 = Select(t=w400, s=w357, f=w399) -> (s? t:f=w401:dbl)
                n292 = Select(t=w358, s=w357, f=w359) -> (s? t:f=w356:dbl)
                n293 = call <vilib>:"DAQmx Start Task.vi"("task/channels in"=w454, "error in"=w335) -> ("task out"=w453:refnum<k21>, "error out"=w452:errorcluster)  [unwired: 12 in]
                n294 = while {
                  shift-right: [w603] -> _
                  shift-left: 0.0 -> [w607]
                  shift-right: [w602] -> _
                  shift-left: _ -> [w601]
                  tunnel: [w597] -> w465
                  shift-right: [w513] -> _
                  shift-left: FALSE ("Manual pause") -> [w596]
                  tunnel: [w593] -> w460
                  tunnel: [w592] -> w346
                  tunnel: [w591] -> w345
                  tunnel: ["Stop"] -> w466
                  tunnel: w453 -> [w579]
                  tunnel: w452 -> [w578]
                  tunnel: [w505] -> w462
                  tunnel: [w584] -> w459
                  tunnel: [w575] -> w451
                  tunnel: [w574] -> w450
                  tunnel: w449 -> [w573]
                  tunnel: w448 -> [w572]
                  tunnel: "Sweep enabled" -> [w571]
                  tunnel: w437 -> [w570]
                  tunnel: w436 -> [w558]
                  tunnel: [w569] -> w435
                  tunnel: [w555] -> w434
                  tunnel: w432 -> [w562]
                  tunnel: w412 -> [w561]
                  tunnel: w406 -> [w553]
                  tunnel: w401 -> [w520]
                  tunnel: w398 -> [w534]
                  tunnel: w388 -> [w532]
                  tunnel: w386 -> [w530]
                  tunnel: w385 -> [w529]
                  shift-right: [w524] -> w374
                  shift-left: sgl[][] [] -> [w523]
                  tunnel: w356 -> [w518]
                  tunnel: w351 -> [w512]
                  tunnel: w350 -> [w511]
                  i -> [w517]
                  stop <- w604 stop-if-true
                  w583 = u32 0 ("milliseconds to wait")
                  w587 = 100.0 ("x")
                  n295 = Random Number (0-1)() -> (number: 0 to 1=w563:dbl)
                  n296 = Greater?(x=w517, y=u32 1 ("millisecond multiple")) -> (0:w515:bool)
                  n297 = local read "Line progress"() -> (w595:u8)
                  n298 = local write "Total progress"(w534) -> ()
                  n299 = local read "Manual pause"() -> (w513:bool)
                  n300 = local read "Milling para"() -> (w564:T1)
                  n301 = local read "FIB PID on"() -> (w550:bool)
                  n302 = local read "Beam blanked"() -> (w549:bool)
                  n303 = local read "Manual pause"() -> (w527:bool)
                  n304 = local read "FIB PID measured"() -> (w528:u8)
                  n305 = local read "Manual pause"() -> (w590:bool)
                  n306 = Equal To 0?(x=w517) -> (x = 0?=w552:bool)
                  n307 = Tick Count (ms)() -> (millisecond timer value=w602:u32)
                  n308 = local read "Line milling time (s)"() -> (w599:sgl)
                  n309 = Subtract(x=w602, y=w601) -> (x-y=w546:u32)
                  n310 = Wait Until Next ms Multiple(millisecond multiple=u32 100) -> ()  [unwired: 1 out]
                  n311 = expression code="x/1000"("FIB bit size (nm)") -> (w567:dbl)
                  n312 = Unbundle By Name(w564) -> ("FIB FOV (um)"=w565:sgl)
                  n313 = expression code="x*2-1"(w563) -> (w560:dbl)
                  n314 = Not(x=w549) -> (.not. x?=w548:bool)
                  n315 = Not(x=w527) -> (.not. x?=w526:bool)
                  n316 = Select(t=w520, s=w515, f=w518) -> (s? t:f=w519:dbl)
                  n317 = Build Array(w595, w534) -> (w594:u8[])
                  n318 = local read "FIB PID reset"() -> (w536:bool)
                  n319 = Compound Arithmetic op=OR(w590, w552) -> (w600:bool)
                  n320 = Not Equal?(x=w513, y=w596) -> (x != y?=w551:bool)
                  n321 = Compound Arithmetic op=AND(w550, w548, w526) -> (w533:bool)
                  n322 = shared-variable ".\\Zeiss Library.lvlib\\Milling Progress"(w594) -> ()  [unwired: 1 in, 1 out]
                  n323 = Select(t=u32 0, s=w600, f=w546) -> (s? t:f=w605:u32)
                  n324 = Compound Arithmetic op=MULTIPLY(w599, 1000.0 ("y"), w553) -> (w582:dbl)
                  n325 = Not(x=w513) -> (.not. x?=w535:bool)
                  n326 = Divide(x=w567, y=w565) -> (x/y=w568:dbl)
                  n327 = Add(x=w582, y=w583) -> (x+y=w581:dbl)
                  n328 = Add(x=w605, y=w607) -> (x+y=w603:dbl)
                  n329 = local read "Machine Type"() -> (w514:u8)
                  n330 = Compound Arithmetic op=MULTIPLY(w568, w560, w561) -> (w559:dbl)
                  n331 = local read "FIB PID target"() -> (w537:sgl)
                  n332 = local read "FIB PID target slope"() -> (w542:sgl)
                  n333 = Divide(x=w546, y=u32 1000) -> (x/y=w547:dbl)
                  n334 = Divide(x=w603, y=w581) -> (x/y=w543:dbl)
                  n335 = Greater Or Equal?(x=w603, y=w581) -> (x >= y?=w507:bool)
                  n336 = And(x=w535, y=w536) -> (x .and. y?=w525:bool)
                  n337 = expression code="(x-0.5)*2"(w543) -> (w541:dbl)
                  n338 = local read "ActiveX Container"() -> (w580:refnum<k7>)
                  n339 = case shown="True" w552 {
                    tunnel: [_ w720] -> w593
                    tunnel: w583 -> [_ w719]
                    tunnel: w580 -> [_ w718]
                    frame False {
                    }
                    frame True {
                      n340 = stacked-sequence {
                        tunnel: [_ w725] -> w720
                        tunnel: w719 -> [w721 _]
                        tunnel: w718 -> [_ w722]
                        frame #0 {
                          n341 = Wait (ms)(milliseconds to wait=w721) -> ()  [unwired: 1 out]
                        }
                        frame #1 {
                          w723 = FALSE ("Beam blanked")
                          n342 = local read "Beam blank"() -> (w724:tag)
                          n343 = local write "Beam blanked"(w723) -> ()
                          n344 = call "FIB beam blank.vi"("ActiveX Container"=w722, "Beam blanked"=w723, "lines"=w724) -> ("error out"=w725:errorcluster)  [unwired: 2 in]
                        }
                      }
                    }
                  }
                  n345 = Sign(1:w537) -> (0:w509:sgl)
                  n346 = Multiply(x=-1.0, y=w509) -> (x*y=w508:dbl)
                  n347 = case shown="True" w551 {
                    tunnel: [_ w728] -> w597
                    tunnel: w513 -> [_ w727]
                    tunnel: w514 -> [_ w726]
                    frame False {
                    }
                    frame True {
                      n348 = case shown="False" w727 {
                        tunnel: [w730 w766] -> w728
                        tunnel: w726 -> [w729 w764]
                        frame False {
                          n349 = stacked-sequence {
                            tunnel: [_ _ _ _ _ w761] -> w730
                            tunnel: w729 -> [w731 w744 _ _ _ _]
                            frame #0 {
                              n350 = case shown="2" w731 {
                                frame 0, Default {
                                }
                                frame 1 {
                                w734 = TRUE ("Initialization")
                                n351 = local read "COM port"() -> (w735:refnum<visa-resource-name>)
                                n352 = local read "Milling mode"() -> (w733:T2)
                                n353 = case shown="\"FIB\"" w733 {
                                tunnel: ["edx 0" ("SEM command") "edx 1" ("SEM command")] -> w732
                                frame "SEM + FIB", Default {
                                }
                                frame "FIB" {
                                }
                                }
                                n354 = call "Remcon32 command.vi"("Close session"=w734, "Initialization"=w734, "SEM command"=w732, "COM port in"=w735) -> ()  [unwired: 4 in, 4 out]
                                }
                                frame 2 {
                                n355 = local read "ActiveX Container"() -> (w742:refnum<k7>)
                                n356 = call "SmartSEM Remote API FIB mode.vi"("FIB mode"=T5."Ext", "ActiveX Container"=w742) -> ("error out"=w738:errorcluster, "reference out"=w739:refnum<k7>)  [unwired: 8 in]
                                n357 = invoke class="_EMApi" method="Set"(reference=w739, error in=w738, "lpszParam"="DP_FIB_BLANKED", "vValue"=sgl 0.0) -> ()  [unwired: 1 in, 5 out]
                                }
                              }
                            }
                            frame #1 {
                              n358 = case shown="1" w744 {
                                frame 0, Default {
                                }
                                frame 1 {
                                w746 = TRUE ("Initialization")
                                n359 = local read "COM port"() -> (w747:refnum<visa-resource-name>)
                                n360 = local read "Milling mode"() -> (w745:T2)
                                n361 = call "FIB mode.vi"("Close session"=w746, "Initialization"=w746, "FIB mode"=w745, "COM port in"=w747) -> ()  [unwired: 6 in, 2 out]
                                }
                              }
                            }
                            frame #2 {
                              n362 = local read "FIB HW Config"() -> (w751:T4)
                              n363 = Unbundle By Name(w751) -> ("Shutter Drive"=w750:tag)
                              n364 = call "Shutter Swing V3.vi"("Shutter Drive"=w750, "Damping"="Damping", "Shutter close"=TRUE) -> ("Fail #"=w753:u8, "SEM shutter status"=w754:string, "Color Box"=w749:u32)  [unwired: 2 in, 4 out]
                              n365 = property on="SEM shutter status" class="Str"("Text.BGColor"=w749) -> ()  [unwired: 2 in, 2 out]
                              n366 = local write "SEM shutter status"(w754) -> ()
                              n367 = local write "Fail #"(w753) -> ()
                              n368 = Wait (ms)(milliseconds to wait=u32 100) -> ()  [unwired: 1 out]
                            }
                            frame #3 {
                              n369 = local read "Ext scan"() -> (w757:tag)
                              n370 = call "FIB ext scan.vi"("Ext on"=TRUE, "FIB Ext Scan"=w757) -> ()  [unwired: 9 in, 1 out]
                            }
                            frame #4 {
                              n371 = Wait (ms)(milliseconds to wait=u32 100) -> ()  [unwired: 1 out]
                            }
                            frame #5 {
                              w760 = FALSE ("Beam blanked")
                              n372 = local read "ActiveX Container"() -> (w759:refnum<k7>)
                              n373 = local read "Beam blank"() -> (w762:tag)
                              n374 = local write "Beam blanked"(w760) -> ()
                              n375 = call "FIB beam blank.vi"("ActiveX Container"=w759, "Beam blanked"=w760, "lines"=w762) -> ("error out"=w761:errorcluster)  [unwired: 2 in]
                            }
                          }
                        }
                        frame True {
                          w765 = TRUE ("Beam blanked")
                          n376 = local read "ActiveX Container"() -> (w763:refnum<k7>)
                          n377 = local read "Beam blank"() -> (w767:tag)
                          n378 = case shown="1" w764 {
                            frame 0, Default {
                            }
                            frame 1 {
                              w768 = TRUE ("Initialization")
                              n379 = local read "COM port"() -> (w770:refnum<visa-resource-name>)
                              n380 = call "Remcon32 command.vi"("Close session"=w768, "Initialization"=w768, "SEM command"="edx 0", "COM port in"=w770) -> ()  [unwired: 4 in, 4 out]
                            }
                            frame 2 {
                            }
                          }
                          n381 = call "FIB beam blank.vi"("ActiveX Container"=w763, "Beam blanked"=w765, "lines"=w767) -> ("error out"=w766:errorcluster)  [unwired: 2 in]
                          "Beam blanked" <- w765
                        }
                      }
                    }
                  }
                  n382 = local read "Beam blanked"() -> (w521:bool)
                  n383 = call <vilib>:"DAQmx Is Task Done.vi"("task/channels in"=w579, "error in"=w578) -> ("task out"=w592:refnum<k21>, "error out"=w591:errorcluster)  [unwired: 2 in, 10 out]
                  n384 = Compound Arithmetic op=MULTIPLY(w509, w542, w541) -> (w540:dbl)
                  n385 = Increment(x=w540) -> (x+1=w539:dbl)
                  n386 = Multiply(x=w537, y=w539) -> (x*y=w538:dbl)
                  n387 = case shown="True" w533 {
                    tunnel: w547 -> [_ w627]
                    tunnel: [0.0 ("Feedback") w626] -> w554
                    tunnel: w519 -> [_ w625]
                    tunnel: w538 -> [_ w624]
                    tunnel: w528 -> [_ w623]
                    tunnel: w525 -> [_ w622]
                    tunnel: w512 -> [_ w621]
                    tunnel: w511 -> [_ w620]
                    tunnel: w508 -> [_ w619]
                    frame False {
                      n388 = local write "FIB PID FB array"(dbl[] [] ("array")) -> ()
                    }
                    frame True {
                      n389 = stacked-sequence {
                        tunnel: w627 -> [_ w662 _]
                        tunnel: [_ w658 _] -> w626
                        tunnel: w625 -> [_ w654 _]
                        tunnel: w624 -> [_ w636 _]
                        tunnel: w623 -> [_ w650 _]
                        tunnel: w622 -> [w628 _ w698]
                        tunnel: w621 -> [_ w634 _]
                        tunnel: w620 -> [_ w633 _]
                        tunnel: w619 -> [_ w632 _]
                        frame #0 {
                          n390 = case shown="True" w628 {
                            frame False {
                            }
                            frame True {
                              w629 = 0.0 ("FIB PID feedback")
                              n391 = local write "FIB PID feedback"(w629) -> ()
                              n392 = local write "FIB PID feedback mean"(w629) -> ()
                            }
                          }
                        }
                        frame #1 {
                          (unwired) 0.5 ("Measured upper limit")
                          n393 = local read "FIB PID I"() -> (w645:sgl)
                          n394 = local read "FIB PID P"() -> (w648:sgl)
                          n395 = shared-variable ".\\Zeiss Library.lvlib\\Logs"() -> (w659:sgl[])  [unwired: 1 in, 1 out]
                          n396 = case shown="0, Default" w650 {
                            tunnel: [w668 100.0 ("Measured upper limit") 100.0 ("Measured upper limit") 100.0 ("Measured upper limit") 100.0 ("Measured upper limit")] -> w651
                            tunnel: [1 ("index") 2 ("index") 3 ("index") 4 ("index") 4 ("index")] -> w643
                            tunnel: [w663 1.0 ("Measured upper limit") -1.0 ("Measured upper limit") -1.0 ("Measured upper limit") -1.0 ("Measured upper limit")] -> w646
                            tunnel: [500.0 ("Measured upper limit") 0.1 ("Measured upper limit") 500.0 ("Measured upper limit") 0.1 ("Measured upper limit") 0.1 ("Measured upper limit")] -> w639
                            tunnel: w636 -> [w667 w672 w677 w685 _]
                            tunnel: [w667 w672 w677 w684 w693] -> w635
                            tunnel: w634 -> [w665 _ _ w683 w692]
                            tunnel: w632 -> [w663 _ _ _ _]
                            frame 0, Default {
                              n397 = expression code="x/2"(w665) -> (w664:sgl)
                              n398 = Greater Than 0?(x=w667) -> (x > 0?=w666:bool)
                              n399 = Select(t=500.0 ("Measured upper limit"), s=w666, f=w664) -> (s? t:f=w668:dbl)
                            }
                            frame 1 {
                            }
                            frame 2 {
                            }
                            frame 3 {
                              n400 = In Range and Coerce(upper limit=w683, x=w685, lower limit=0.0 ("Measured upper limit")) -> (coerced(x)=w684:dbl)  [unwired: 1 out]
                            }
                            frame 4 {
                              n401 = shared-variable ".\\Zeiss Library.lvlib\\FIB mill target by spec. I"() -> (w691:sgl)  [unwired: 1 in, 1 out]
                              n402 = In Range and Coerce(upper limit=w692, x=w691, lower limit=0.0 ("Measured upper limit")) -> (coerced(x)=w693:dbl)  [unwired: 1 out]
                            }
                          }
                          n403 = Index Array(array=w659, index #1=2 ("index"), index #2=w643) -> (element #1=w641:sgl, element #2=w644:sgl)
                          n404 = Multiply(x=w645, y=w646) -> (x*y=w647:dbl)
                          n405 = Multiply(x=w648, y=w646) -> (x*y=w649:dbl)
                          n406 = Greater?(x=w641, y=w633) -> (0:w640:bool)
                          n407 = local read "FIB PID FB array"() -> (w630:dbl[])
                          n408 = Select(t=-100.0 ("Measured upper limit"), s=w640, f=w639) -> (s? t:f=w638:dbl)
                          n409 = Array Size(array=w630) -> (size(s)=w631:i32)
                          n410 = call "PID Feedback.vi"("Measured"=w644, "Proportional"=w649, "Integral"=w647, "Measured upper limit"=w651, "Measured lower limit"=w638, "Target"=w635, "Feedback offset if measured exceed limits"=w654, "Cycle time"=w662, "Feedback low limit"=-1.0 ("Low limit"), "Feedback high limit"=1.0 ("High limit")) -> ("Feedback"=w658:dbl)  [unwired: 4 in, 1 out]
                          "FIB PID feedback" <- w658
                          n411 = Build Array (concatenate)(w630, w658) -> (w653:dbl[])
                          "FIB PID FB array" <- w653
                          n412 = expression code="x-4"(w631) -> (w652:i32)
                          n413 = Array Subset(array=w653, index=4, length=w652) -> (w656:dbl[])
                          n414 = call-poly <vilib>:"Mean.vi"("X"=w656) -> ("mean"=→"FIB PID feedback mean":dbl)  [unwired: 1 out]
                        }
                        frame #2 {
                          n415 = case shown="True" w698 {
                            frame False {
                            }
                            frame True {
                              n416 = local write "FIB PID reset"(FALSE ("FIB PID reset")) -> ()
                            }
                          }
                        }
                      }
                    }
                  }
                  n417 = Compound Arithmetic op=ADD(w559, w562, w554) -> (w531:dbl)
                  n418 = In Range and Coerce(upper limit=w530, x=w531, lower limit=w529) -> (coerced(x)=w522:dbl)  [unwired: 1 out]
                  "Z voltage RT" <- w522
                  n419 = case shown="True" w521 {
                    tunnel: [w610 w613] -> w524
                    tunnel: w523 -> [w609 w613]
                    tunnel: w522 -> [w608 _]
                    frame False {
                      n420 = shared-variable ".\\Zeiss Library.lvlib\\Logs"() -> (w611:sgl[])  [unwired: 1 in, 1 out]
                      n421 = Build Array (concatenate)(w611, w608) -> (w612:dbl[])
                      n422 = Build Array (concatenate)(w609, w612) -> (w610:dbl[][])
                    }
                    frame True {
                    }
                  }
                  n423 = case shown="True" w571 {
                    tunnel: [FALSE ("status") w707] -> w576
                    tunnel: [w702 w706] -> w575
                    tunnel: [w701 w705] -> w574
                    tunnel: w573 -> [w702 w704]
                    tunnel: w572 -> [w701 w703]
                    frame False {
                    }
                    frame True {
                      n424 = call <vilib>:"DAQmx Is Task Done.vi"("task/channels in"=w704, "error in"=w703) -> ("task out"=w706:refnum<k21>, "error out"=w705:errorcluster)  [unwired: 2 in, 10 out]
                      n425 = Unbundle By Name(w705) -> ("status"=w707:bool)
                    }
                  }
                  n426 = shared-variable ".\\Zeiss Library.lvlib\\Milling Z Voltage RT"(w522) -> ()  [unwired: 1 in, 1 out]
                  n427 = Multiply(x=w587, y=w543) -> (x*y=w588:dbl)
                  n428 = In Range and Coerce(upper limit=w587, x=w588, lower limit=0.0) -> (coerced(x)=w586:dbl)  [unwired: 1 out]
                  n429 = Unbundle By Name(w591) -> ("status"=w557:bool)
                  n430 = local write "Line progress"(w586) -> ()
                  n431 = call-poly <vilib>:"DAQmx Write.vi"("task/channels in"=w570, "data"=w522, "error in"=w558) -> ("task out"=w569:refnum<k21>, "error out"=w555:errorcluster)  [unwired: 1 in, 10 out]
                  n432 = case shown="True" w533 {
                    tunnel: w522 -> [_ w616]
                    tunnel: w532 -> [_ w615]
                    frame False {
                    }
                    frame True {
                      n433 = Subtract(x=w616, y=w615) -> (x-y=w614:dbl)
                      n434 = local write "FIB PID on offset"(w614) -> ()
                    }
                  }
                  n435 = Unbundle By Name(w555) -> ("status"=w556:bool)
                  n436 = Or(x=w557, y=w556) -> (x .or. y?=w505:bool)
                  n437 = Or(x=w505, y=w507) -> (x .or. y?=w506:bool)
                  n438 = case shown="True" w506 {
                    tunnel: [_ w711] -> w584
                    tunnel: [FALSE ("Beam blanked") w710] -> w577
                    tunnel: w580 -> [_ w709]
                    frame False {
                    }
                    frame True {
                      n439 = stacked-sequence {
                        tunnel: [w715 _ _] -> w711
                        tunnel: [_ _ TRUE ("Beam blanked")] -> w710
                        tunnel: w709 -> [w712 _ _]
                        frame #0 {
                          w713 = TRUE ("Beam blanked")
                          n440 = local read "Beam blank"() -> (w714:tag)
                          n441 = local write "Beam blanked"(w713) -> ()
                          n442 = call "FIB beam blank.vi"("ActiveX Container"=w712, "Beam blanked"=w713, "lines"=w714) -> ("error out"=w715:errorcluster)  [unwired: 2 in]
                        }
                        frame #1 {
                          n443 = Wait (ms)(milliseconds to wait=u32 10) -> ()  [unwired: 1 out]
                        }
                        frame #2 {
                        }
                      }
                    }
                  }
                  n444 = Compound Arithmetic op=OR(w577, w576, w505, "Stop") -> (w604:bool)
                }
                n445 = local read "FIB X coil"() -> (w338:tag)
                n446 = call <vilib>:"DAQmx Clear Task.vi"("task in"=w346, "error in"=w345) -> ("error out"=w337:errorcluster)  [unwired: 13 out]
                n447 = call <vilib>:"DAQmx Clear Task.vi"("task in"=w435, "error in"=w434) -> ("error out"=w433:errorcluster)  [unwired: 13 out]
                n448 = case shown="False" "Sweep enabled" {
                  tunnel: [w471 w474] -> w457
                  tunnel: w451 -> [_ w473]
                  tunnel: w450 -> [w471 w472]
                  frame False {
                  }
                  frame True {
                    n449 = call <vilib>:"DAQmx Clear Task.vi"("task in"=w473, "error in"=w472) -> ("error out"=w474:errorcluster)  [unwired: 13 out]
                  }
                }
                n450 = Merge Errors(w465, w337, w433, w459, w460, w457) -> (w347:errorcluster)
                "error out" <- w347
                n451 = call-poly <vilib>:"DAQmx Create Virtual Channel.vi"("physical channels"=w338, "error in"=w337) -> ("task out"=w339:refnum<k21>, "error out"=w336:errorcluster)  [unwired: 7 in, 5 out]
                n452 = Transpose 2D Array(2D array=w374) -> (transposed array=w375:dbl[][])
                n453 = call <vilib>:"General Error Handler.vi"("error in (no error)"=w347) -> ()  [unwired: 10 in, 5 out]
                n454 = for {
                  tunnel: [w469] -> w362 mode=indexing
                  tunnel: w375 -> [w468] mode=indexing
                  n455 = call-poly <vilib>:"Basic Averaged DC-RMS.vi"("signal in"=w468) -> ("DC value"=w469:dbl)  [unwired: 7 in, 3 out]
                }
                n456 = call-poly <vilib>:"DAQmx Write.vi"("task/channels in"=w339, "data"=-8.0, "error in"=w336) -> ("task out"=w341:refnum<k21>, "error out"=w340:errorcluster)  [unwired: 1 in, 10 out]
                n457 = call "FM Gen Pulse for FIB-SEM.vi"("WatchDog Mode"="WatchDog Mode", "error in"=w347, "State Value"=i16 3) -> ()  [unwired: 6 in, 3 out]
                n458 = To Single Precision Float(number=w362) -> (single precision float=w361:sgl[])
                n459 = Index Array(array=w361, index #1=0 ("index"), index #2=1 ("index"), index #3=2 ("index"), index #4=3 ("index"), index #5=4 ("index"), index #6=5 ("index")) -> (element #1=w364:sgl, element #2=w370:sgl, element #3=w369:sgl, element #4=w368:sgl, element #5=w367:sgl, element #6=w360:sgl)
                n460 = shared-variable ".\\Zeiss Library.lvlib\\Faraday cup offset"(w364) -> (error out=w333:errorcluster)  [unwired: 1 in]
                n461 = shared-variable ".\\Zeiss Library.lvlib\\Specimen (nA)"(w370, error in=w333) -> (error out=w332:errorcluster)
                n462 = shared-variable ".\\Zeiss Library.lvlib\\Beam Dump 1 (nA)"(w369, error in=w332) -> (error out=w331:errorcluster)
                n463 = shared-variable ".\\Zeiss Library.lvlib\\Beam Dump 2 (nA)"(w368, error in=w331) -> (error out=w330:errorcluster)
                n464 = shared-variable ".\\Zeiss Library.lvlib\\Milling I (nA)"(w367, error in=w330) -> (error out=w329:errorcluster)
                n465 = shared-variable ".\\Zeiss Library.lvlib\\Milling Z Voltage"(w360, error in=w329) -> ()  [unwired: 1 out]
                n466 = call <vilib>:"DAQmx Start Task.vi"("task/channels in"=w341, "error in"=w340) -> ("task out"=w343:refnum<k21>, "error out"=w344:errorcluster)  [unwired: 12 in]
                n467 = call <vilib>:"DAQmx Clear Task.vi"("task in"=w343, "error in"=w344) -> ()  [unwired: 14 out]
              }
              frame True {
                w771 = TRUE
              }
            }
          }
          frame #3 {
            n468 = local read "Sweep enabled"() -> (w772:bool)
            n469 = case shown="True" w772 {
              frame False {
              }
              frame True {
                n470 = local read "Shutter Drive"() -> (w776:tag)
                n471 = call-poly <vilib>:"DAQmx Create Virtual Channel.vi"("physical channels"=w776) -> ("task out"=w774:refnum<k21>, "error out"=w773:errorcluster)  [unwired: 13 in]
                n472 = call-poly <vilib>:"DAQmx Write.vi"("task/channels in"=w774, "data"=dbl[] [0.0, 0.0, 0.0, 0.0], "error in"=w773) -> ("task out"=w778:refnum<k21>, "error out"=w779:errorcluster)  [unwired: 1 in, 10 out]
                n473 = call <vilib>:"DAQmx Clear Task.vi"("task in"=w778, "error in"=w779) -> ("error out"=w775:errorcluster)  [unwired: 13 out]
                n474 = call <vilib>:"General Error Handler.vi"("error in (no error)"=w775) -> ()  [unwired: 10 in, 5 out]
                n475 = local write "error out"(w775) -> ()
              }
            }
          }
        }
        n476 = local read "Stop"() -> (w119:bool)
        n477 = Compound Arithmetic op=OR(w122, w126, w132, w119) -> (w123:bool)
      }
      n478 = case shown="True" w88 {
        frame False {
        }
        frame True {
          n479 = local write "Line Paused"(TRUE ("Line Paused")) -> ()
        }
      }
    }
    frame #2 {
      w782 = TRUE ("Beam blanked")
      n480 = local read "Machine Type"() -> (w781:u8)
      n481 = local read "Ext scan"() -> (w784:tag)
      n482 = local read "ActiveX Container"() -> (w780:refnum<k7>)
      n483 = local read "Beam blank"() -> (w786:tag)
      n484 = local write "Stop"(FALSE ("Stop")) -> ()
      n485 = case shown="2" w781 {
        frame 0, Default {
        }
        frame 1 {
        }
        frame 2 {
          n486 = local read "ActiveX Container"() -> (w791:refnum<k7>)
          n487 = call "SmartSEM Remote API set float.vi"("vValue"=sgl 2.0, "lpszParam"="DP_FIB_BLANKER_MODE" ("lpszCommand"), "ActiveX Container"=w791) -> ("error out"=w787:errorcluster, "reference out"=w788:refnum<k7>)  [unwired: 7 in]
          n488 = call "SmartSEM Remote API FIB mode.vi"("error in"=w787, "FIB mode"=T5."SEM", "ActiveX Container"=w788) -> ("error out"=w792:errorcluster, "reference out"=w793:refnum<k7>)  [unwired: 7 in]
          n489 = invoke class="_EMApi" method="Execute"(reference=w793, error in=w792, "lpszCommand"="CMD_FREEZE_ALL") -> ()  [unwired: 1 in, 4 out]
        }
      }
      n490 = local write "Beam blanked"(w782) -> ()
      n491 = call "FIB ext scan.vi"("Ext on"=FALSE ("data"), "FIB Ext Scan"=w784) -> ()  [unwired: 9 in, 1 out]
      n492 = call "FIB beam blank.vi"("ActiveX Container"=w780, "Beam blanked"=w782, "lines"=w786) -> ()  [unwired: 2 in, 1 out]
    }
  }
